vi "Set safety delay.vi"(8 "error in":errorcluster, 10 "Safety delay (Active)":u16(ring) items=["Active", "Over-Ridden"], 11 "VISA resource name":refnum<visa-resource-name>) -> (0 "error out":errorcluster, 3 "VISA resource name out":refnum<visa-resource-name>)   [LabVIEW 2012, in "Datron D4xxx.lvlib"]
doc: "This VI enables/disables instrument safety delay."
uses:
  Datron D4xxx.lvlib
panel:
  out "Error Message":string
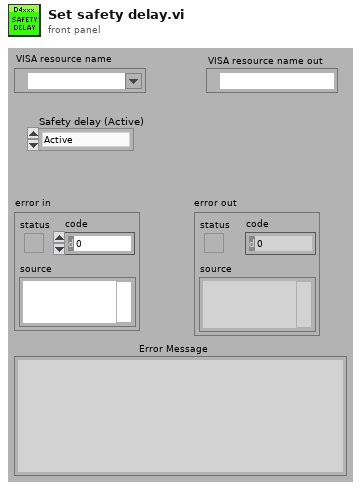
[diagram p1: front panel]
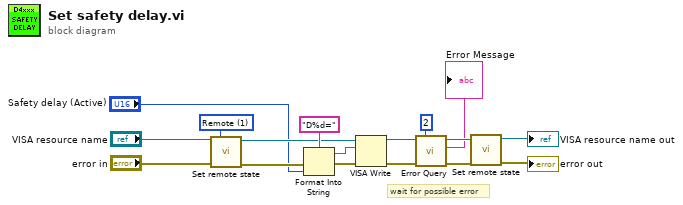
[diagram p0: block diagram]
diagram:
  w4 = u16 1 items=["Local", "Remote", "Default"] ("Remote state")
  # "wait for possible error"
  n1 = call "Set remote state.vi"("error in"="error in", "Remote state"=w4, "VISA resource name"="VISA resource name") -> ("error out"=w7:errorcluster, "VISA resource name out"=w5:refnum<visa-resource-name>)  [unwired: 7 in]
  n2 = Format Into String(format string="D%d=", error in=w7, "Safety delay (Active)") -> (resulting string=w17:string, error out=w16:errorcluster)  [unwired: 1 in]
  n3 = VISA Write(VISA resource name=w5, write buffer=w17, error in (no error)=w16) -> (VISA resource name out=w9:refnum<visa-resource-name>, error out=w10:errorcluster)  [unwired: 1 out]
  n4 = call "Error Query.vi"("error in (no error)"=w10, "Check cycles (11)"=2, "VISA resource name"=w9) -> ("error out"=w14:errorcluster, "Error Message"=→"Error Message":string, "VISA resource name out"=w12:refnum<visa-resource-name>)  [unwired: 5 in, 1 out]
  n5 = call "Set remote state.vi"("error in"=w14, "VISA resource name"=w12) -> ("error out"=→"error out":errorcluster, "VISA resource name out"=→"VISA resource name out":refnum<visa-resource-name>)  [unwired: 8 in]
